vi "Config - Read.vi"(8 "error in (no error)":errorcluster) -> (0 "error out":errorcluster, 3 "Data Records":T1[](array[typedef]))   [LabVIEW 2017]
doc: "Reads from Congifuration DB all data records."
uses:
  Controls/Config Data Record.ctl
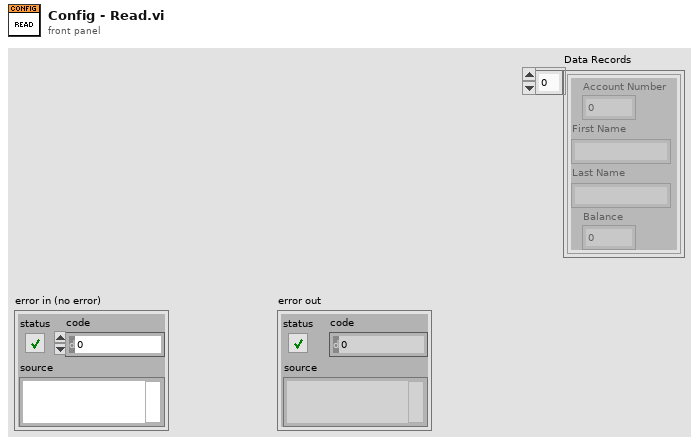
[diagram p1: front panel]
types:
  T1 = typedef "Config Data Record.ctl" = cluster{"Account Number":u32, "First Name":string, "Last Name":string, "Balance":dbl}
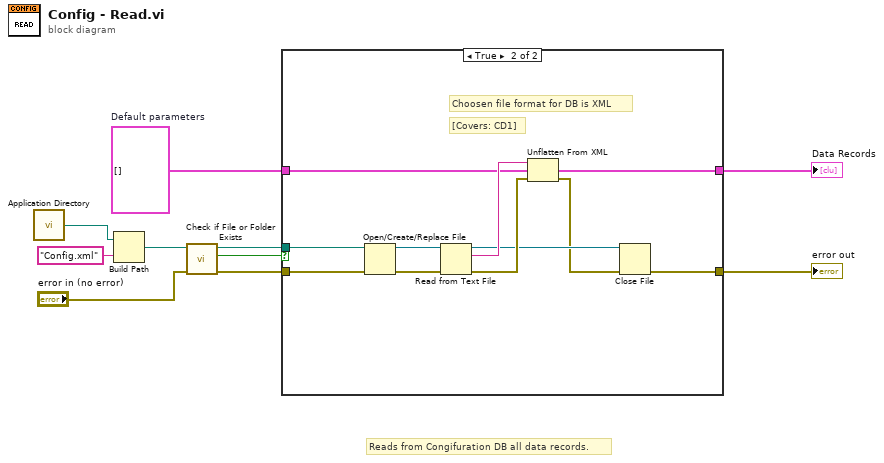
[diagram p0: block diagram]
diagram:
  w3 = T1[] []  # Default parameters
  # "Reads from Congifuration DB all data records."
  n1 = call <vilib>:"Application Directory.vi"() -> ("Application Directory"=w10:path)
  n2 = Build Path(base path=w10, name or relative path="Config.xml") -> (appended path=w8:path)
  n3 = call <vilib>:"Check if File or Folder Exists.vi"("error in (no error)"="error in (no error)", "path"=w8) -> ("error out"=w6:errorcluster, "file or folder exists?"=w7:bool, "dup path"=w5:path)  [unwired: 7 in]
  n4 = case shown="True" w7 {
    tunnel: w6 -> [w11 w23]
    tunnel: w5 -> [_ w22]
    tunnel: w3 -> [w12 w15]
    tunnel: [w11 w14] -> w1
    tunnel: [w12 w13] -> w2
    frame False {
      # "[Covers: CD4]"
      # "IF config.xml not found\nTHEN use default parameters"
    }
    frame True {
      # "[Covers: CD1]"
      # "Choosen file format for DB is XML"
      n5 = Open/Create/Replace File(file path (use dialog)=w22, error in=w23) -> (refnum out=w20:refnum<file>, error out=w21:errorcluster)  [unwired: 4 in, 1 out]
      n6 = Read from Text File(file (use dialog)=w20, error in=w21) -> (refnum out=w17:refnum<file>, text=w19:string, error out=w18:errorcluster)  [unwired: 2 in, 1 out]
      n7 = Unflatten From XML(xml string=w19, type=w15, error in (no error)=w18) -> (value=w13:T1[], error out=w16:errorcluster)
      n8 = Close File(refnum=w17, error in=w16) -> (error out=w14:errorcluster)  [unwired: 1 out]
    }
  }
  "Data Records" <- w2
  "error out" <- w1
